vi "Mixer.ToggleTalkback.vi"   [LabVIEW 2020]
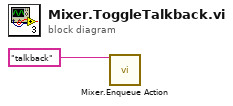
[diagram p0: block diagram]
diagram:
  n1 = call "Mixer.Enqueue Action.vi"("action"="talkback") -> ()  [unwired: 14 in, 1 out]
